vi "Get LLB Methods.vi"(8 "error in (no error)":errorcluster {"code" format="Error %.0f"}, 11 "LLB Documentation In":refnum<class "LLB Documentation.lvclass">) -> (0 "error out":errorcluster {"code" format="Error %.0f"}, 2 "LLB Methods":T1[](array[typedef]), 3 "LLB Documentation Out":refnum<class "LLB Documentation.lvclass">)   [LabVIEW 2023, in "VIDoc Parsing.lvlib" / "LLB Documentation.lvclass"]
uses:
  LLB Documentation.lvclass
  TypeDefs/Method Spec Cluster.ctl
  TypeDefs/VI Type Extended Enum.ctl
  <vilib>/picture/picture.llb/imagedata.ctl
  TypeDefs/Class Dispatch Type Enum.ctl
  TypeDefs/Controls Info Cluster.ctl
  <vilib>/Utility/miscctls.llb/LVKeyTypeDef.ctl
  <vilib>/Utility/miscctls.llb/LVPointTypeDef.ctl
  SubVIs/Structure Reporter/Tree Cluster.ctl
  LLB Documentation.lvclass/LLB Documentation.ctl
  VIDoc Parsing.lvlib
  SubVIs/Structure Reporter/Structure Reporter.lvlib
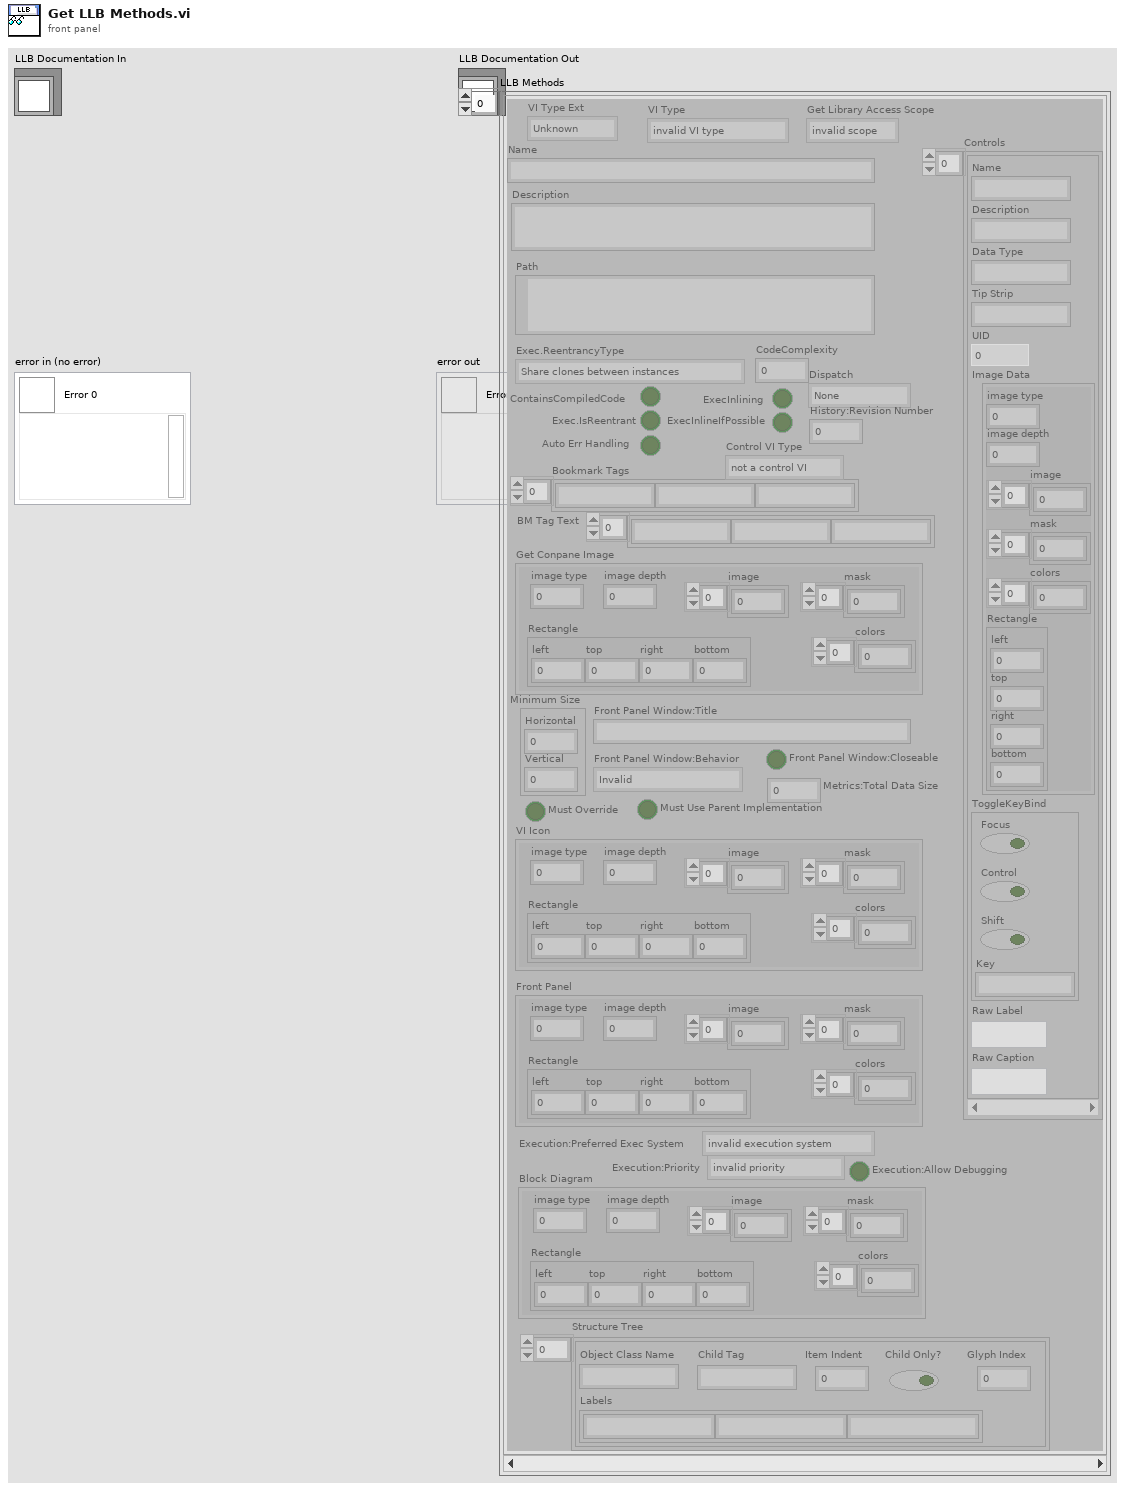
[diagram p1: front panel]
types:
  T1 = typedef "VIDoc Parsing.lvlib/Method Spec Cluster.ctl" = cluster{"VI Type Ext":T2, "Name":string, "Path":path, "Get Conpane Image":T3, "Description":string, "Get Library Access Scope":enum32{"invalid scope", "public", "private", "protected", "community"}, "Dispatch":T4, "ContainsCompiledCode":bool, "Exec.IsReentrant":bool, "Exec.ReentrancyType":enum16{"Share clones between instances", "Preallocate clone for each instance"}, "ExecInlining":bool, "ExecInlineIfPossible":bool, "Auto Err Handling":bool, "CodeComplexity":sgl, "Bookmark Tags":string[], "Control VI Type":enum32{"not a control VI", "control", "typedef", "strict typedef"}, "Controls":T5[], "VI Type":enum32{"invalid VI type", "Standard VI", "Control VI", "Global VI", "Polymorphic VI", "Configuration VI", "SubSystem", "Facade VI", "Method VI", "Statechart Diagram VI"}, "Minimum Size":T7, "Front Panel Window:Title":string, "Front Panel Window:Behavior":enum32{"Invalid", "Default", "Floating", "Floating/Auto-Hide", "Modal"}, "Front Panel Window:Closeable":bool, "Must Override":bool, "Must Use Parent Implementation":bool, "VI Icon":T3, "Front Panel":T3, "History:Revision Number":u32, "Metrics:Total Data Size":u32, "Execution:Allow Debugging":bool, "Execution:Preferred Exec System":enum32{"invalid execution system", "user interface", "standard", "instrument i/o", "data acquisition", "other 1", "other 2", "same as caller"}, "Execution:Priority":enum32{"invalid priority", "background priority", "normal priority", "above normal priority", "high priority", "time critical priority", "subroutine"}, "BM Tag Text":string[], "Block Diagram":T3, "Structure Tree":T8[]}
  T2 = typedef "VIDoc Parsing.lvlib/VI Type Extended Enum.ctl" = enum16{"Unknown", "Class Method", "Class Accessor Get", "Class Accessor Set", "Class Control", "Library Method", "Library Control", "VI", "Control"}
  T3 = typedef "imagedata.ctl" = cluster{"image type":i32, "image depth":i32, "image":u8[], "mask":u8[], "colors":u32[], "Rectangle":cluster{"left":i16, "top":i16, "right":i16, "bottom":i16}}
  T4 = typedef "VIDoc Parsing.lvlib/Class Dispatch Type Enum.ctl" = enum16{"None", "Static", "Dynamic"}
  T5 = typedef "VIDoc Parsing.lvlib/Controls Info Cluster.ctl" = cluster{"Name":string, "Description":string, "Data Type":string, "Tip Strip":string, "UID":i32, "Image Data":T3, "ToggleKeyBind":T6, "Raw Label":string, "Raw Caption":string}
  T6 = typedef "LVKeyTypeDef.ctl" = cluster{"Focus":bool, "Control":bool, "Shift":bool, "Key":string}
  T7 = typedef "LVPointTypeDef.ctl" = cluster{"Horizontal":i16, "Vertical":i16}
  T8 = typedef "VIDoc Parsing.lvlib/Structure Reporter.lvlib/Tree Cluster.ctl" = cluster{"Object Class Name":string, "Labels":string[], "Child Tag":string, "Item Indent":i32, "Child Only?":bool, "Glyph Index":i32}
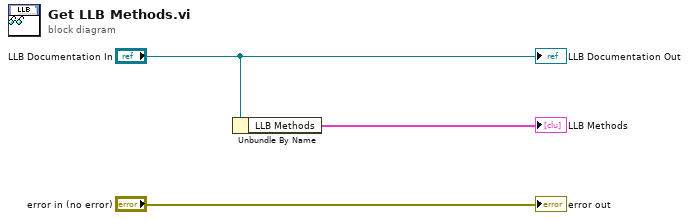
[diagram p0: block diagram]
diagram:
  n1 = Unbundle By Name("LLB Documentation In") -> ("LLB Methods"=→"LLB Methods":T1[])
  "error out" <- "error in (no error)"
  "LLB Documentation Out" <- "LLB Documentation In"
